vi "PrepLineObjectArray_get_and_lock.vi"(8 "error in (no error)":errorcluster) -> (0 "error out":errorcluster, 3 "PrepLineObjArray out":refnum<class "PrepLineObject.lvclass">[](array[class]))   [LabVIEW 2013]
doc: "the VI locks the PreplineObjectArray in order to restrict access to one process only. When the access is locked it returns the most up-to-date PrepLineObject Array from the global variable"
uses:
  Classes/PrepLineObject/PrepLineObject.lvclass
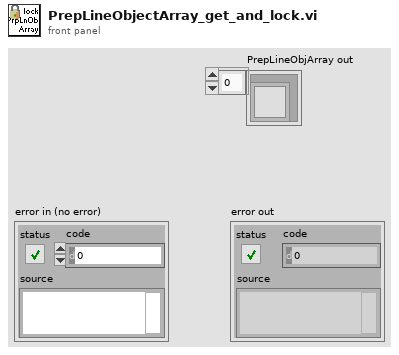
[diagram p1: front panel]
types:
  T1 = typedef "Semaphore RefNum" = refnum<k1>
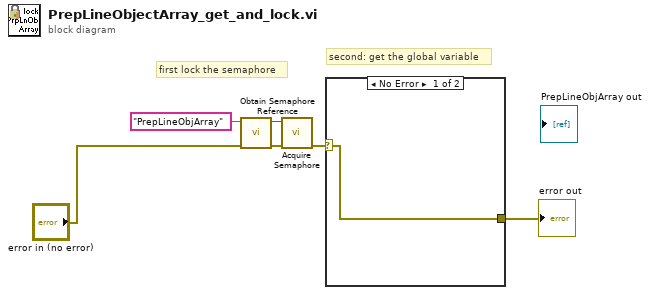
[diagram p0: block diagram]
diagram:
  # "second: get the global variable"
  # "first lock the semaphore"
  n1 = call <vilib>:"Obtain Semaphore Reference.vi"("error in (no error)"="error in (no error)", "name (unnamed)"="PrepLineObjArray") -> ("error out"=w3:errorcluster, "semaphore"=w5:T1)  [unwired: 3 in, 1 out]
  n2 = call <vilib>:"Acquire Semaphore.vi"("error in (no error)"=w3, "semaphore"=w5) -> ("error out"=w2:errorcluster)  [unwired: 3 in, 2 out]
  n3 = case shown="No Error" w2 {
    selector: w2 -> [w7 w8]
    tunnel: [w7 w8] -> w1
    frame No Error {
    }
    frame Error {
    }
  }
  "error out" <- w1
